vi "Untitled 5.vi"() -> ()   [LabVIEW 2025]
panel:
  out "Array":string[][](array[string])
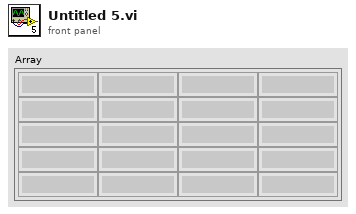
[diagram p1: front panel]
types:
  T1 = cluster{"Module IDs":i32[], "Module Names":string[]}
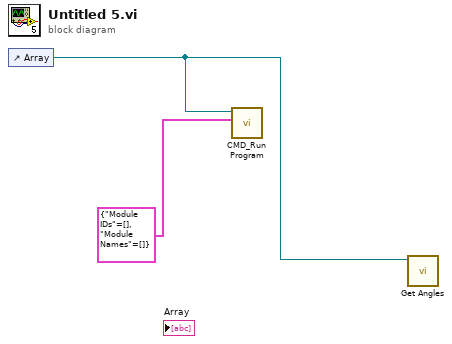
[diagram p0: block diagram]
diagram:
  n1 = control-ref of="Array"() -> (w1:refnum<vi>)
  n2 = call "CMD_Run Program.vi"("Modules"=T1 {"Module IDs"=[], "Module Names"=[]}, "Array in"=w1) -> ()  [unwired: 9 in, 1 out]
  n3 = call "Get Angles.vi"("Array in"=w1) -> ()  [unwired: 9 in, 2 out]
